vi "Periodic Tasks.vi"(8 "error in":errorcluster) -> ()   [LabVIEW 2018]
doc: "This VI runs in parallel to other tasks. It can contain as many user-defined periodic loops as you need. These can carry out PID or other sorts of timed response."
uses:
  Right Motors.ctl
  Left Motors.ctl
  Solenoids.ctl
  <vilib>/Rock Robotics/WPI/Solenoid/WPI_SolenoidValue.ctl
  <vilib>/Rock Robotics/WPI/ThirdParty/Phoenix-LabVIEW/Motor Controller/Controls/CTRE_Phoenix_MotorControl_ControlMode.ctl
  Robot Global Data.vi
  <vilib>/Rock Robotics/WPI/Solenoid/WPI_SolenoidSetEnum.vi
  SwerveLibrary/Huskie Swerve.lvlib
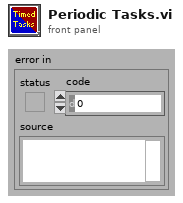
[diagram p1: front panel]
types:
  T1 = typedef "Solenoids.ctl" = enum16{"Solenoid 1", "Solenoid 2", "Solenoid 3", "Solenoid 4"}
  T2 = typedef "Left Motors.ctl" = enum16{"Left Motors 1", "Left Motors 2", "Left Motors 3"}
  T3 = typedef "Right Motors.ctl" = enum16{"Right Motors 1", "Right Motors 2", "Right Motors 3"}
  T4 = typedef "WPI_MotorControlDeviceRef.ctl" = cluster{"DeviceStatus":errorcluster, "Type":T5, "PWM":cluster{"PWM Channel":T6, "DeadBand":T7}, "CAN":cluster{"Device Number":u8, "SetOutput VI Ref":variant, "GetOutput VI Ref":variant, "Enable VI Ref":variant, "Disable VI Ref":variant, "Data":variant}, "Invert":bool, "DIO PWM":cluster{"PWM \"Enable\" Channel":T6, "DIOChannel":T8, "PWM Rate":dbl}}
  T5 = typedef "WPI_MotorControlType.ctl" = enum16{"PWM", "CAN", "DIO PWM"}
  T6 = typedef "FPGA_DIOPWMChannel.ctl" = enum8{"PWM 0", "PWM 1", "PWM 2", "PWM 3", "PWM 4", "PWM 5", "PWM 6", "PWM 7", "PWM 8", "PWM 9", "PWM MXP 0", "PWM MXP 1", "PWM MXP 2", "PWM MXP 3", "PWM MXP 4", "PWM MXP 5", "PWM MXP 6", "PWM MXP 7", "PWM MXP 8", "PWM MXP 9", "Invalid"}
  T7 = typedef "WPI_PWMDeadband.ctl" = cluster{"Name":string, "maxPositivePwm":i32, "minPositivePwm":i32, "centerPwm":i32, "maxNegativePwm":i32, "minNegativePwm":i32, "angularRange":u16}
  T8 = typedef "FPGA_DIOChannel.ctl" = enum8{"DIO 0", "DIO 1", "DIO 2", "DIO 3", "DIO 4", "DIO 5", "DIO 6", "DIO 7", "DIO 8", "DIO 9", "DIO MXP 0", "DIO MXP 1", "DIO MXP 2", "DIO MXP 3", "DIO MXP 4", "DIO MXP 5", "DIO MXP 6", "DIO MXP 7", "DIO MXP 8", "DIO MXP 9", "DIO MXP 10", "DIO MXP 11", "DIO MXP 12", "DIO MXP 13", "DIO MXP 14", "DIO MXP 15", "SPI Port CS1", "SPI Port CS2", "SPI Port CS3", "SPI Port MISO", "SPI Port MOSI", "Invalid"}
  T9 = typedef "WPI_SolenoidDevRef.ctl" = cluster{"DevStatus":errorcluster, "Pneumatics Control Module":u8, "Forward Solenoid Channel":T10, "Reverse Solenoid Channel":T10}
  T10 = typedef "WPI_SolenoidChannel.ctl" = enum8{"Solenoid 0", "Solenoid 1", "Solenoid 2", "Solenoid 3", "Solenoid 4", "Solenoid 5", "Solenoid 6", "Solenoid 7", "Invalid"}
  T11 = typedef "WPI_SolenoidValue.ctl" = enum16{"Off", "On", "Forward", "Reverse"}
  T12 = typedef "CTRE_Phoenix_MotorControl_ControlMode.ctl" = u16
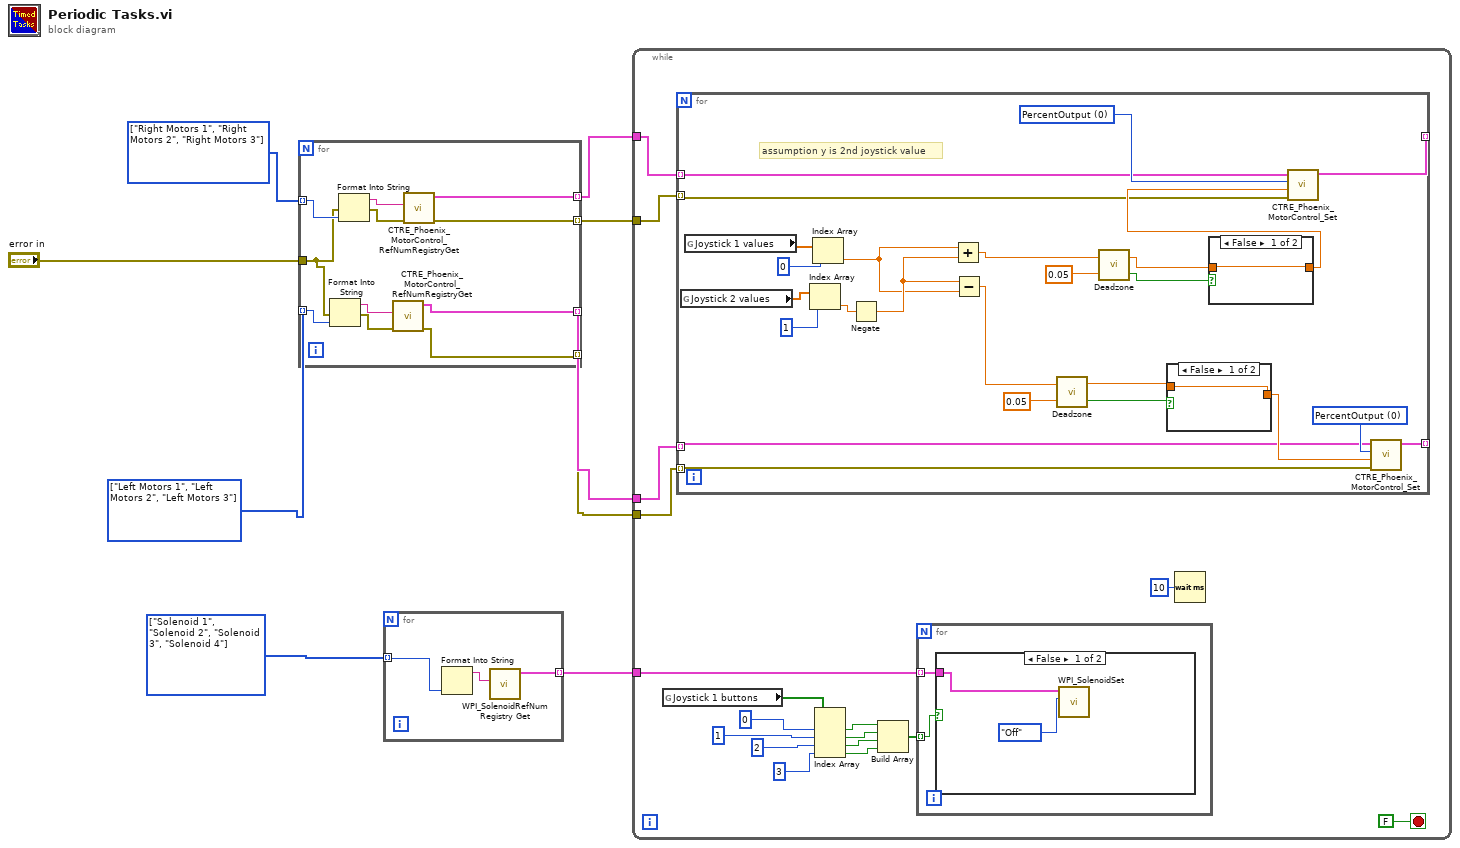
[diagram p0: block diagram]
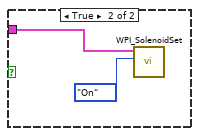
[diagram p2: hidden frame]
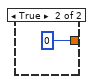
[diagram p3: hidden frame]
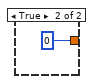
[diagram p4: hidden frame]
diagram:
  w2 = T1[] [enum."Solenoid 1", enum."Solenoid 2", enum."Solenoid 3", enum."Solenoid 4"] items=["Solenoid 1", "Solenoid 2", "Solenoid 3", "Solenoid 4"] ("Array")
  w8 = T2[] [enum."Left Motors 1", enum."Left Motors 2", enum."Left Motors 3"] items=["Left Motors 1", "Left Motors 2", "Left Motors 3"]
  w9 = T3[] [enum."Right Motors 1", enum."Right Motors 2", enum."Right Motors 3"] items=["Right Motors 1", "Right Motors 2", "Right Motors 3"]
  n1 = for {
    tunnel: w9 -> [w20] mode=indexing
    tunnel: w8 -> [w18] mode=indexing
    tunnel: [w16] -> w7 mode=indexing
    tunnel: [w15] -> w6 mode=indexing
    tunnel: "error in" -> [w14]
    tunnel: [w11] -> w4 mode=indexing
    tunnel: [w10] -> w3 mode=indexing
    n2 = Format Into String(error in=w14, w18) -> (resulting string=w17:string, error out=w13:errorcluster)  [unwired: 2 in]
    n3 = Format Into String(error in=w14, w20) -> (resulting string=w19:string, error out=w12:errorcluster)  [unwired: 2 in]
    n4 = call <vilib>:"CTRE_Phoenix_MotorControl_RefNumRegistryGet.vi"("error in (no error)"=w13, "refnum name"=w17) -> ("error out"=w11:errorcluster, "PhoenixMotorControlDevRef"=w16:T4)  [unwired: 8 in]
    n5 = call <vilib>:"CTRE_Phoenix_MotorControl_RefNumRegistryGet.vi"("error in (no error)"=w12, "refnum name"=w19) -> ("error out"=w10:errorcluster, "PhoenixMotorControlDevRef"=w15:T4)  [unwired: 8 in]
  }
  n6 = for {
    tunnel: w2 -> [w22] mode=indexing
    tunnel: [w21] -> w1 mode=indexing
    n7 = Format Into String(w22) -> (resulting string=w23:string)  [unwired: 3 in, 1 out]
    n8 = call <vilib>:"WPI_SolenoidRefNum Registry Get.vi"("refnum name"=w23) -> ("SolenoidDevRef"=w21:T9)  [unwired: 9 in, 1 out]
  }
  n9 = while {
    tunnel: w7 -> [w40]
    tunnel: w6 -> [w39]
    tunnel: w4 -> [w36]
    tunnel: w3 -> [w24]
    tunnel: w1 -> [w25]
    stop <- FALSE stop-if-true
    n10 = global read "Robot Global Data.vi" "Joystick 1 buttons"() -> (w35:bool[])
    n11 = for {
      tunnel: [w71] -> _ mode=indexing
      tunnel: [w70] -> _ mode=indexing
      tunnel: w40 -> [w50] mode=indexing
      tunnel: w39 -> [w67] mode=indexing
      tunnel: w36 -> [w60] mode=indexing
      tunnel: w24 -> [w54] mode=indexing
      w68 = T12 0 items=["PercentOutput"=0, "Position"=1, "Velocity"=2, "Current"=3, "Follower"=5, "MotionProfile"=6, "MotionMagic"=7, "MotionMagicArc"=8, "MotionProfileArc"=10, "Disabled"=15] ("Control Mode")
      w69 = T12 0 items=["PercentOutput"=0, "Position"=1, "Velocity"=2, "Current"=3, "Follower"=5, "MotionProfile"=6, "MotionMagic"=7, "MotionMagicArc"=8, "MotionProfileArc"=10, "Disabled"=15] ("Control Mode")
      # "assumption y is 2nd joystick value"
      n12 = global read "Robot Global Data.vi" "Joystick 2 values"() -> (w66:dbl[])
      n13 = global read "Robot Global Data.vi" "Joystick 1 values"() -> (w65:dbl[])
      n14 = Index Array(array=w66, index=1) -> (element=w62:dbl)
      n15 = Index Array(array=w65, index=0) -> (element=w59:dbl)
      n16 = Negate(x=w62) -> (-x=w61:dbl)
      n17 = Add(x=w59, y=w61) -> (x+y=w58:dbl)
      n18 = Subtract(x=w61, y=w59) -> (x-y=w52:dbl)
      n19 = call "Deadzone.vi"("Deadzone"=0.05, "Value"=w52) -> ("Inside Deadzone?"=w49:bool, "Numeric"=w48:dbl)
      n20 = call "Deadzone.vi"("Deadzone"=0.05, "Value"=w58) -> ("Inside Deadzone?"=w56:bool, "Numeric"=w47:dbl)
      n21 = case shown="False" w49 {
        tunnel: [w72 0] -> w51
        tunnel: w48 -> [w72 _]
        frame False {
        }
        frame True {
        }
      }
      n22 = case shown="False" w56 {
        tunnel: [w74 0] -> w55
        tunnel: w47 -> [w74 _]
        frame False {
        }
        frame True {
        }
      }
      n23 = call <vilib>:"CTRE_Phoenix_MotorControl_Set.vi"("error in (no error)"=w54, "Output"=w55, "Control Mode"=w69, "PhoenixMotorControlDevRef"=w67) -> ("PhoenixMotorControlDevRef"=w71:T4)  [unwired: 6 in, 1 out]
      n24 = call <vilib>:"CTRE_Phoenix_MotorControl_Set.vi"("error in (no error)"=w60, "Output"=w51, "Control Mode"=w68, "PhoenixMotorControlDevRef"=w50) -> ("PhoenixMotorControlDevRef"=w70:T4)  [unwired: 6 in, 1 out]
    }
    n25 = Index Array(array=w35, index #1=0 ("index"), index #2=1 ("index"), index #3=2 ("index"), index #4=3 ("index")) -> (element #1=w30:bool, element #2=w29:bool, element #3=w28:bool, element #4=w27:bool)
    n26 = Build Array(w30, w29, w28, w27) -> (w26:bool[])
    n27 = for {
      tunnel: w26 -> [w42] mode=indexing
      tunnel: w25 -> [w41] mode=indexing
      n28 = case shown="False" w42 {
        tunnel: w41 -> [w44 w46]
        frame False {
          n29 = call-poly <vilib>:"WPI_SolenoidSet.vi"("Value"=WPI_SolenoidValue."Off", "SolenoidDevRef"=w44) -> ()  [unwired: 8 in, 2 out]
        }
        frame True {
          n30 = call-poly <vilib>:"WPI_SolenoidSet.vi"("Value"=WPI_SolenoidValue."On", "SolenoidDevRef"=w46) -> ()  [unwired: 8 in, 2 out]
        }
      }
    }
    n31 = Wait (ms)(milliseconds to wait=10) -> ()  [unwired: 1 out]
  }
